vi "Graphics.vi"() -> ()   [LabVIEW 2020]
panel:
  out "Waveform Chart":cluster{dbl, dbl, dbl}(graph)
  in  "Stop Button":bool
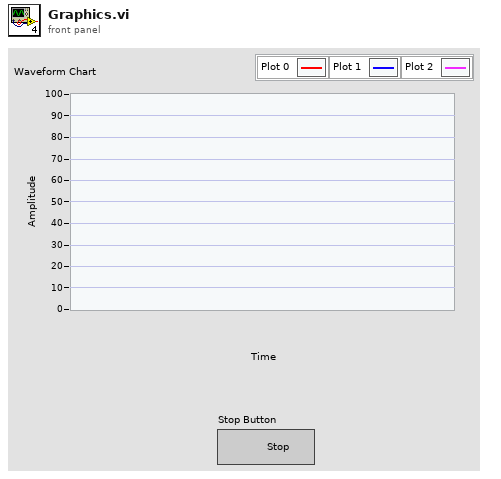
[diagram p1: front panel]
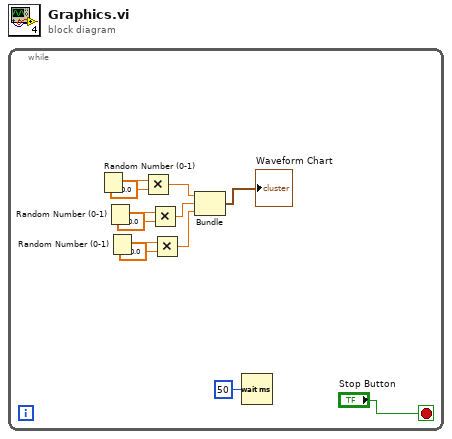
[diagram p0: block diagram]
diagram:
  n1 = while {
    stop <- "Stop Button" stop-if-true
    n2 = Random Number (0-1)() -> (number: 0 to 1=w10:dbl)
    n3 = Random Number (0-1)() -> (number: 0 to 1=w8:dbl)
    n4 = Random Number (0-1)() -> (number: 0 to 1=w2:dbl)
    n5 = Multiply(x=w10, y=100.0) -> (x*y=w5:dbl)
    n6 = Multiply(x=w8, y=100.0) -> (x*y=w6:dbl)
    n7 = Multiply(x=w2, y=100.0) -> (x*y=w1:dbl)
    n8 = Bundle(w5, w6, w1) -> (→"Waveform Chart":cluster{dbl, dbl, dbl})  [unwired: 1 in]
    n9 = Wait (ms)(milliseconds to wait=u32 50) -> ()  [unwired: 1 out]
  }
